vi "Config Average.vi"(0 "VISA resource name":refnum<visa-resource-name>, 5 "Average Type (0: OFF)":u16(ring) items=["OFF", "Linear", "Exponent"], 7 "Constant (0: 8)":u16(ring) items=["8", "16", "32", "64"], 11 "error in (no error)":errorcluster) -> (4 "VISA resource name out":refnum<visa-resource-name>, 15 "error out":errorcluster)   [LabVIEW 2013, in "Yokogawa WT200 Series.lvlib"]
doc: "This VI sends the averaging function commands to the WT200 Series."
uses:
  <instrlib>/Yokogawa WT200 Series/Yokogawa WT200 Series.lvlib
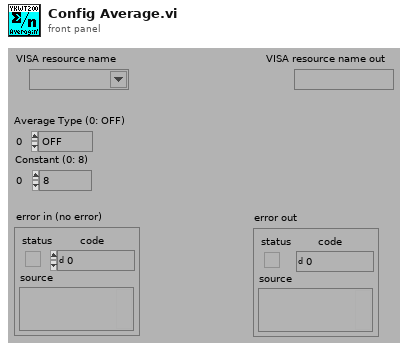
[diagram p1: front panel]
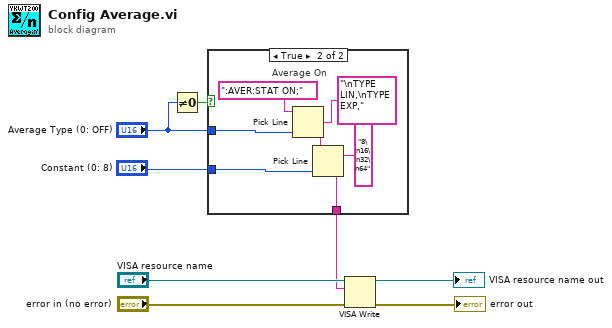
[diagram p0: block diagram]
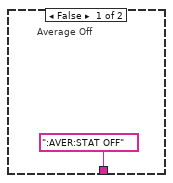
[diagram p2: hidden frame]
diagram:
  n1 = Not Equal To 0?(x="Average Type (0: OFF)") -> (x != 0?=w7:bool)
  n2 = case shown="True" w7 {
    tunnel: [":AVER:STAT OFF" w16] -> w1
    tunnel: "Constant (0: 8)" -> [_ w14]
    tunnel: "Average Type (0: OFF)" -> [_ w10]
    frame False {
      # "Average Off"
    }
    frame True {
      # "Average On"
      n3 = Pick Line(string ("")=":AVER:STAT ON;", multi-line string="\nTYPE LIN,\nTYPE EXP,", line index=w10) -> (output string=w13:string)
      n4 = Pick Line(string ("")=w13, multi-line string="8\n16\n32\n64", line index=w14) -> (output string=w16:string)
    }
  }
  n5 = VISA Write(VISA resource name="VISA resource name", write buffer=w1, error in (no error)="error in (no error)") -> (VISA resource name out=→"VISA resource name out":refnum<visa-resource-name>, error out=→"error out":errorcluster)  [unwired: 1 out]
